vi "Write Position.vi"(8 "error in (no error)":errorcluster, 9 "Position":T1, 10 "Session In":refnum<class "Session.lvclass">, 11 "PCF8574 I2C LCD I in":refnum<class "PCF8574 I2C LCD.lvclass">) -> (0 "error out":errorcluster, 2 "Session Out":refnum<class "Session.lvclass">, 3 "PCF8574 I2C LCD I out":refnum<class "PCF8574 I2C LCD.lvclass">)   [LabVIEW 2020, in "CTI-Peripheral.lvlib" / "PCF8574 I2C LCD.lvclass"]
uses:
  PCF8574 I2C LCD.lvclass
  Character LCD/Position.ctl
  CTI/Session/Session.lvclass
  HD44780 LCD/Command.ctl
  HD44780 LCD/HD44780 LCD.lvlib
  Character LCD/Char LCD.lvclass
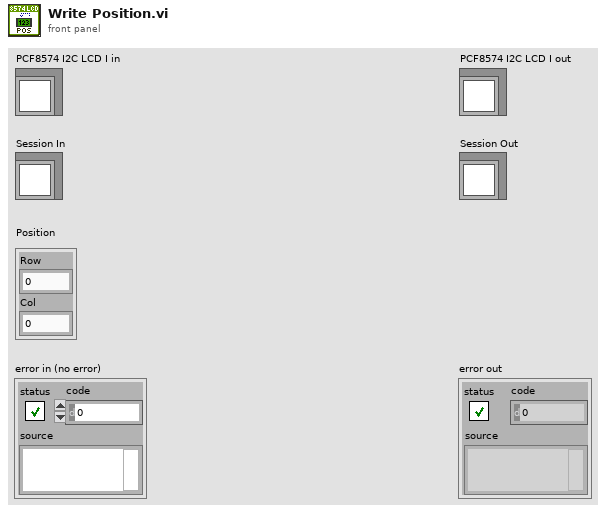
[diagram p1: front panel]
types:
  T1 = typedef "CTI-Peripheral.lvlib/Char LCD.lvclass/Position.ctl" = cluster{"Row":u8, "Col":u8}
  T2 = typedef "CTI-Peripheral.lvlib/HD44780 LCD.lvlib/Command.ctl" = enum16{"ClearDisplay", "ReturnHome", "EntryModeSet", "DisplayControl", "CursorShift", "FunctionSet", "SetCGRamAddr", "SetDDRamAddr"}
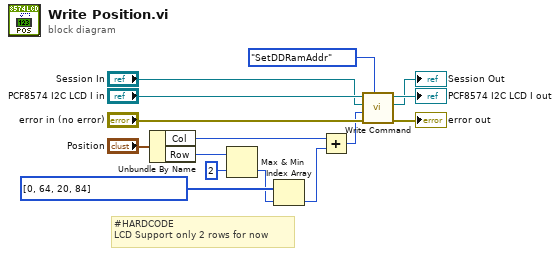
[diagram p0: block diagram]
diagram:
  # "#HARDCODE\nLCD Support only 2 rows for now"
  n1 = Unbundle By Name("Position") -> ("Col"=w11:u8, "Row"=w14:u8)
  n2 = Max & Min(x=w14, y=u8 2) -> (min(x,y)=w12:u8)  [unwired: 1 out]
  n3 = Index Array(array=u8[] [0, 64, 20, 84], index=w12) -> (element=w10:u8)
  n4 = Add(x=w11, y=w10) -> (x+y=w4:u8)
  n5 = call "Write Command.vi"("Command"=Command."SetDDRamAddr", "error in (no error)"="error in (no error)", "Value (0)"=w4, "Session In"="Session In", "PCF8574 I2C LCD in"="PCF8574 I2C LCD I in") -> ("error out"=→"error out":errorcluster, "Session Out"=→"Session Out":refnum<class "Session.lvclass">, "PCF8574 I2C LCD out"=→"PCF8574 I2C LCD I out":refnum<class "PCF8574 I2C LCD.lvclass">)  [unwired: 4 in]
